vi "Array-Subtract First.vi"(4 "Y":dbl[](array[numeric])) -> (1 "Y - mean(Y)":dbl[](array[numeric]))   [LabVIEW 2020]
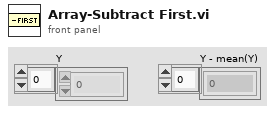
[diagram p1: front panel]
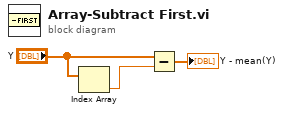
[diagram p0: block diagram]
diagram:
  n1 = Index Array(array="Y") -> (element=w1:dbl)  [unwired: 1 in]
  n2 = Subtract(x="Y", y=w1) -> (x-y=→"Y - mean(Y)":dbl[])
